vi "WayPointCheckoff.vi"(0 "Desired location":T3, 7 "Checkoff Buffer\n(meters)":dbl, 9 "Timeout Buffer\n(meters)":dbl, 11 "Timeout Time\n(seconds)":dbl) -> (6 "Checked Off?":bool=TRUE, 10 "Timed Out?":bool=TRUE)   [LabVIEW 2012]
doc: "Lyra Silverwolf 11/13"
uses:
  cRIO_Code/Data/TypeDefs/UTM Location.ctl
  cRIO_Code/Data/TypeDefs/ocuWaypoint.ctl
  cRIO_Code/Data/TypeDefs/Waypoints List.ctl
  cRIO_Code/Logic/Classes/Waypoint/Waypoint.lvclass
panel:
  in  "GPS Location":T1 {"UTM Location"."North" format="%#_10f"; "UTM Location"."East" format="%#_8f"}
  in  "stop":bool
  # "This is the lengh of time the boat has to check off the waypoint once it is within the timeout buffer"
  # "The boat must be\nwithin this distance\nto the waypoint to \ncheck it off"
  # "This is a secondary distance within which the timeout time begins to count down. The existance of this timeout buffer ensures that the boat does not get stuck circling a waypoint that it will never reach."
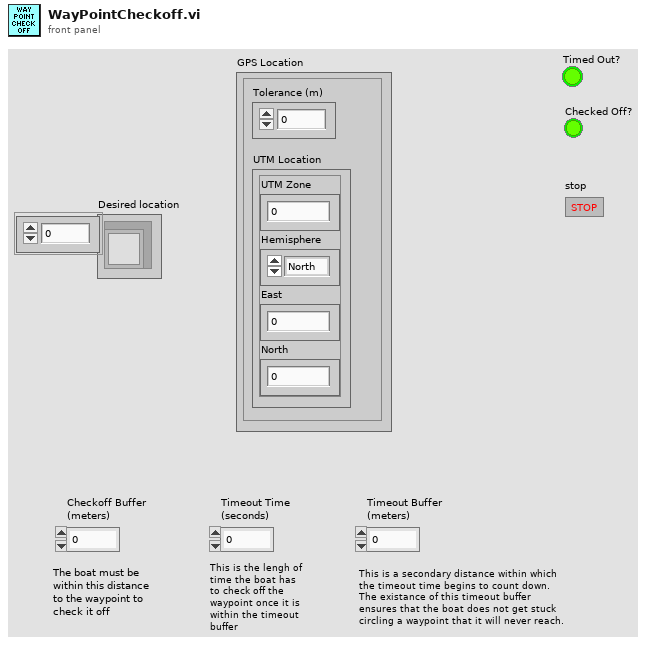
[diagram p1: front panel]
types:
  T1 = typedef "ocuWaypoint.ctl" = cluster{"Tolerance (m)":dbl, "UTM Location":T2}
  T2 = typedef "UTM Location.ctl" = cluster{"UTM Zone":dbl, "Hemisphere":enum16{"North", "South"}, "East":dbl, "North":dbl}
  T3 = typedef "Waypoints List.ctl" = refnum<class "Waypoint.lvclass">[]
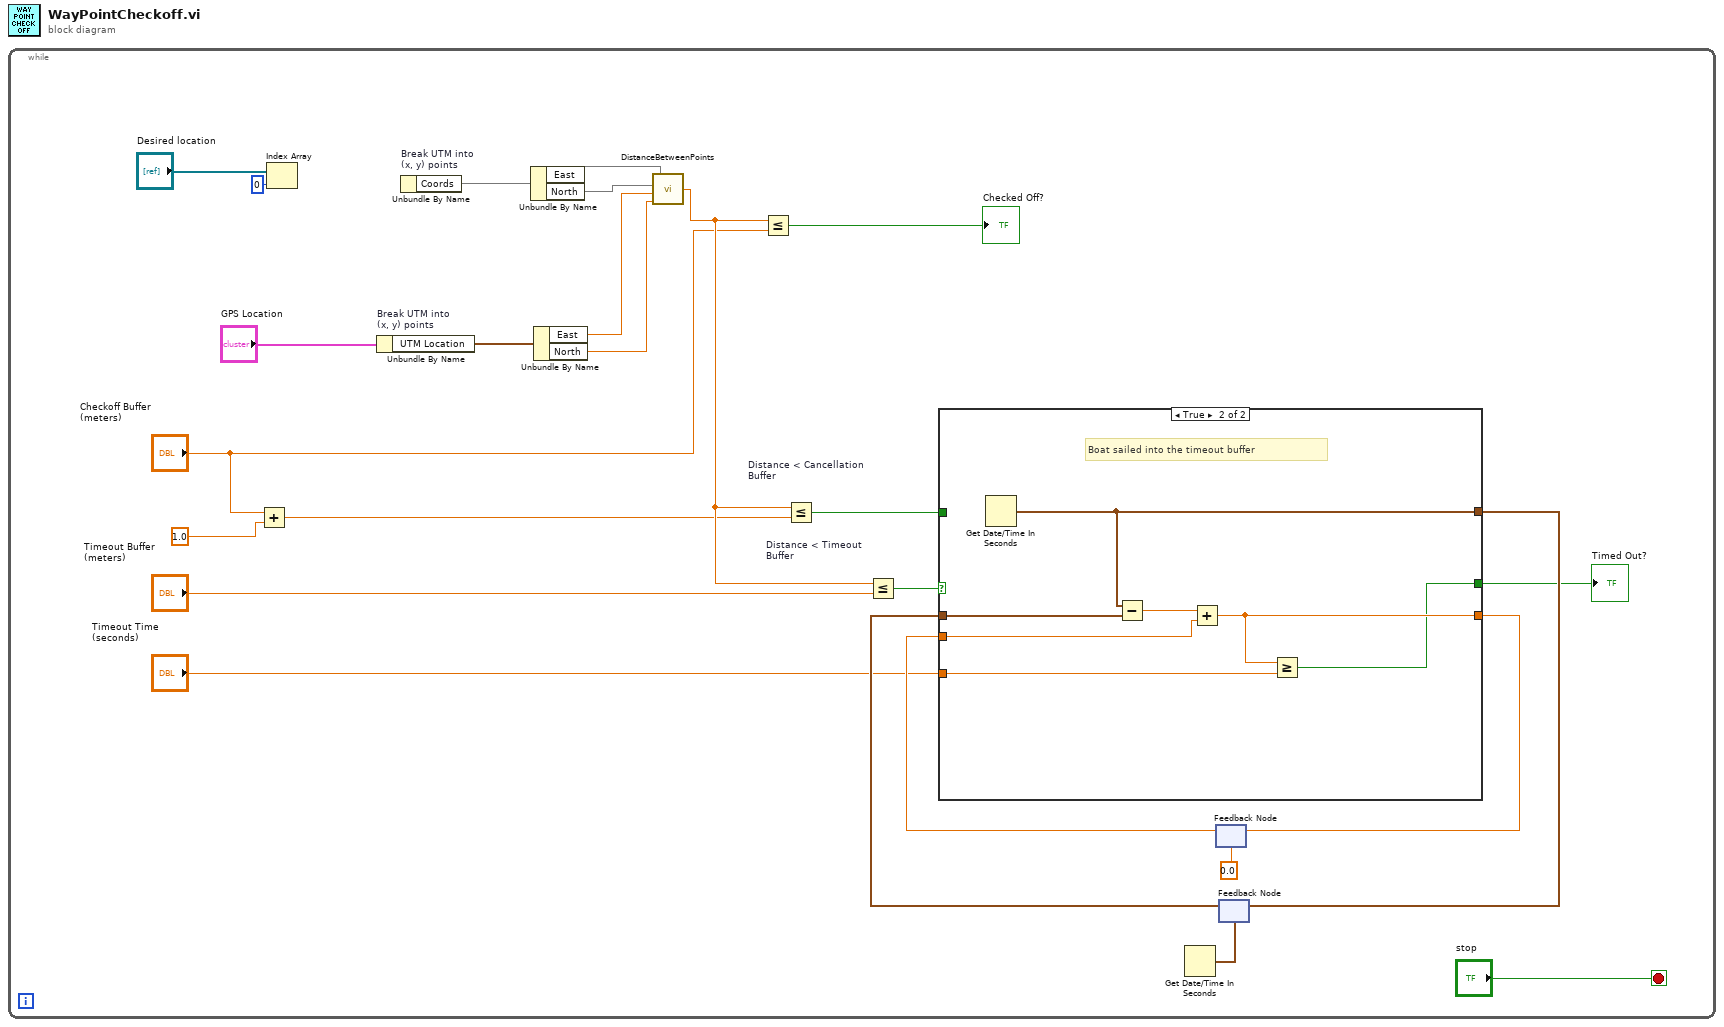
[diagram p0: block diagram]
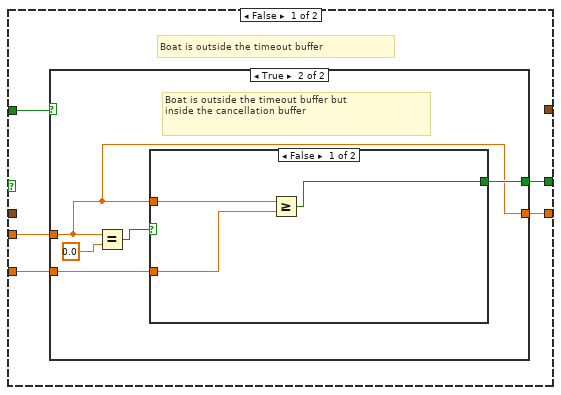
[diagram p2: hidden frame]
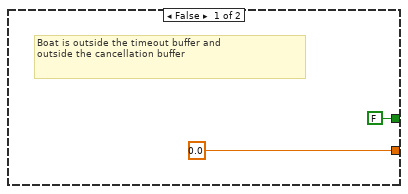
[diagram p3: hidden frame]
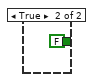
[diagram p4: hidden frame]
diagram:
  n1 = while {
    stop <- "stop" stop-if-true
    n2 = Add(x="Checkoff Buffer\n(meters)", y=1.0) -> (x+y=w10:dbl)
    n3 = Index Array(array="Desired location", index=0) -> ()  [unwired: 1 out]
    n4 = Unbundle By Name "Break UTM into\n(x, y) points"("GPS Location") -> ("UTM Location"=w25:T2)
    n5 = Unbundle By Name "Break UTM into\n(x, y) points"() -> ("Coords"=w26)  [unwired: 1 in]
    n6 = Unbundle By Name(w26) -> ("East"=w24, "North"=w23)
    n7 = Unbundle By Name(w25) -> ("East"=w22:dbl, "North"=w21:dbl)
    n8 = call "DistanceBetweenPoints.vi"("coordinate 2\nnorth"=w21, "coordinate 2\neast"=w22, "coordinate 1\nnorth"=w23, "coordinate 1\neast"=w24) -> ("Numeric"=w20:dbl)
    n9 = Less Or Equal?(x=w20, y="Checkoff Buffer\n(meters)") -> (x <= y?=→"Checked Off?":bool)
    n10 = Less Or Equal? "Distance < Cancellation\nBuffer"(x=w20, y=w10) -> (x <= y?=w16:bool)
    n11 = Less Or Equal? "Distance < Timeout \nBuffer"(x=w20, y="Timeout Buffer\n(meters)") -> (x <= y?=w18:bool)
    n12 = Get Date/Time In Seconds() -> (seconds since 1Jan1904=w7:timestamp)
    n13 = feedback #1(0.0) -> (w13:dbl)
    n14 = feedback #2(w7) -> (w17:timestamp)
    n15 = case shown="True" w18 {
      tunnel: w17 -> [_ w48]
      tunnel: w16 -> [w31 _]
      tunnel: [_ w49] -> w15
      tunnel: w13 -> [w30 w46]
      tunnel: [w29 w44] -> w14
      tunnel: "Timeout Time\n(seconds)" -> [w28 w45]
      tunnel: [w27 w43] -> w4
      frame False {
        # "Boat is outside the timeout buffer"
        n16 = case shown="True" w31 {
          tunnel: w30 -> [_ w34]
          tunnel: [0.0 w34] -> w29
          tunnel: w28 -> [_ w36]
          tunnel: [FALSE w35] -> w27
          frame False {
            # "Boat is outside the timeout buffer and \noutside the cancellation buffer"
          }
          frame True {
            # "Boat is outside the timeout buffer but \ninside the cancellation buffer"
            n17 = Equal?(x=w34, y=0.0) -> (x = y?=w38:bool)
            n18 = case shown="False" w38 {
              tunnel: w34 -> [w41 _]
              tunnel: w36 -> [w40 _]
              tunnel: [w39 FALSE] -> w35
              frame False {
                n19 = Greater Or Equal?(x=w41, y=w40) -> (x >= y?=w39:bool)
              }
              frame True {
              }
            }
          }
        }
      }
      frame True {
        # "Boat sailed into the timeout buffer"
        n20 = Get Date/Time In Seconds() -> (seconds since 1Jan1904=w49:timestamp)
        n21 = Subtract(x=w49, y=w48) -> (x-y=w47:dbl)
        n22 = Add(x=w47, y=w46) -> (x+y=w44:dbl)
        n23 = Greater Or Equal?(x=w44, y=w45) -> (x >= y?=w43:bool)
      }
    }
    "Timed Out?" <- w4
    n24 = feedback-in #1(w14) -> ()
    n25 = feedback-in #2(w15) -> ()
  }
